vi "Get LabVIEW Application Context Reference by Name.vi"(8 "error in (no error)":errorcluster, 11 "Context Name":string) -> (0 "error out":errorcluster, 3 "Application out":refnum<vi>)   [LabVIEW 2020]
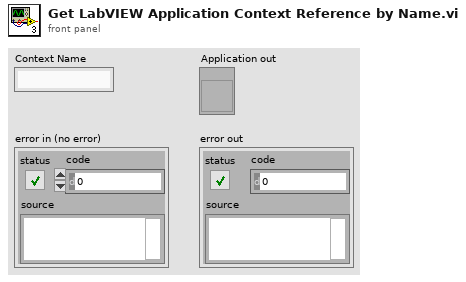
[diagram p1: front panel]
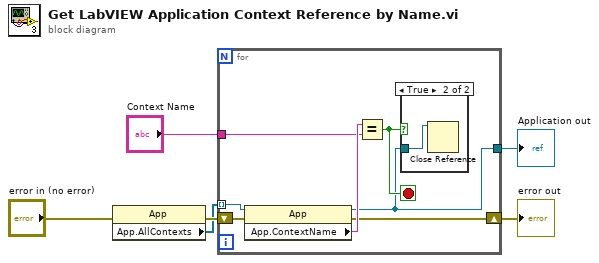
[diagram p0: block diagram]
diagram:
  n1 = property class="App"(error in="error in (no error)") -> (error out=w3:errorcluster, "App.AllContexts"=w1:refnum<vi>[])  [unwired: 1 in, 1 out]
  n2 = for {
    tunnel: w1 -> [w13] mode=indexing
    tunnel: "Context Name" -> [w11]
    shift-right: [w9] -> w6
    shift-left: w3 -> [w10]
    tunnel: [w7] -> w5
    stop <- w8 stop-if-true
    n3 = property class="App"(reference=w13, error in=w10) -> (reference out=w7:refnum<vi>, error out=w9:errorcluster, "App.ContextName"=w12:string)
    n4 = Equal?(x=w12, y=w11) -> (x = y?=w8:bool)
    n5 = case shown="True" w8 {
      tunnel: w7 -> [_ w14]
      frame False {
      }
      frame True {
        n6 = Close Reference(reference=w14) -> ()  [unwired: 1 in, 1 out]
      }
    }
  }
  "error out" <- w6
  "Application out" <- w5
